vi "Date String to Time Stamp.vi"(11 "Date String":string) -> (2 "Time Stamp":timestamp)   [LabVIEW 2021]
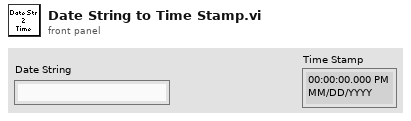
[diagram p1: front panel]
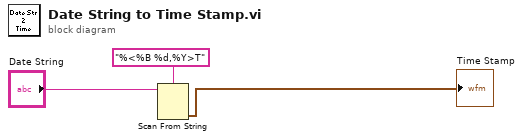
[diagram p0: block diagram]
diagram:
  n1 = Scan From String(format string="%<%B %d,%Y>T", input string="Date String") -> (output 1=→"Time Stamp":timestamp)  [unwired: 3 in, 3 out]
